vi "simulate regional(s).vi"   [LabVIEW 2009]
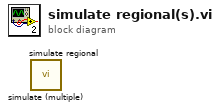
[diagram p0: block diagram]
diagram:
  n1 = call "simulate (multiple).vi"() -> ()  [unwired: 3 in, 2 out]
  n2 = call "simulate regional.vi"() -> ()  [unwired: 3 in, 2 out]
